vi "Sensirion SHT25 - VISA test.vi"() -> ()   [LabVIEW 2012]
uses:
  Sensirion SHT25 - measurement resolution.ctl
panel:
  in  "Reset":bool
  in  "resolution":T1 items=["RH 12, T 14"=0, "RH 8, T 12"=1, "RH 10, T 13"=128, "RH 11, T 11"=129]
  out "user register":u8 format="%08b"
  out "IO pins (initially)":string
  out "Data Chart":cluster{"temperature":dbl, "humidity":dbl}(graph)
  out "temperature":dbl format="%.2f"
  out "humidity":dbl format="%.2f"
  in  "Stop":bool
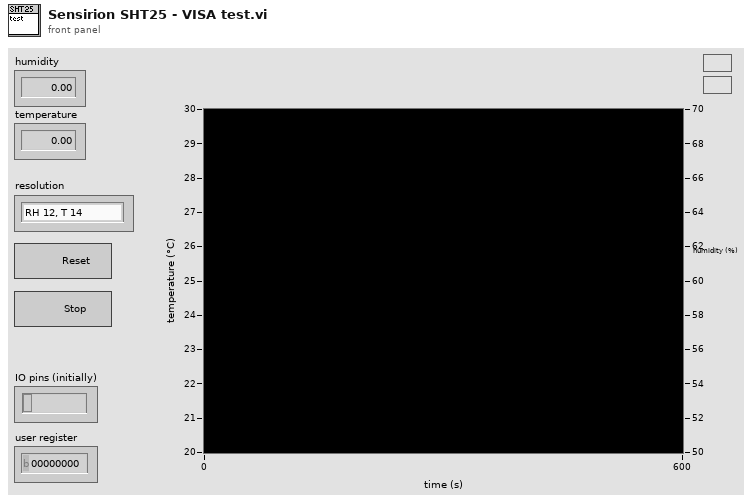
[diagram p1: front panel]
types:
  T1 = typedef "Sensirion SHT25 - measurement resolution.ctl" = u8
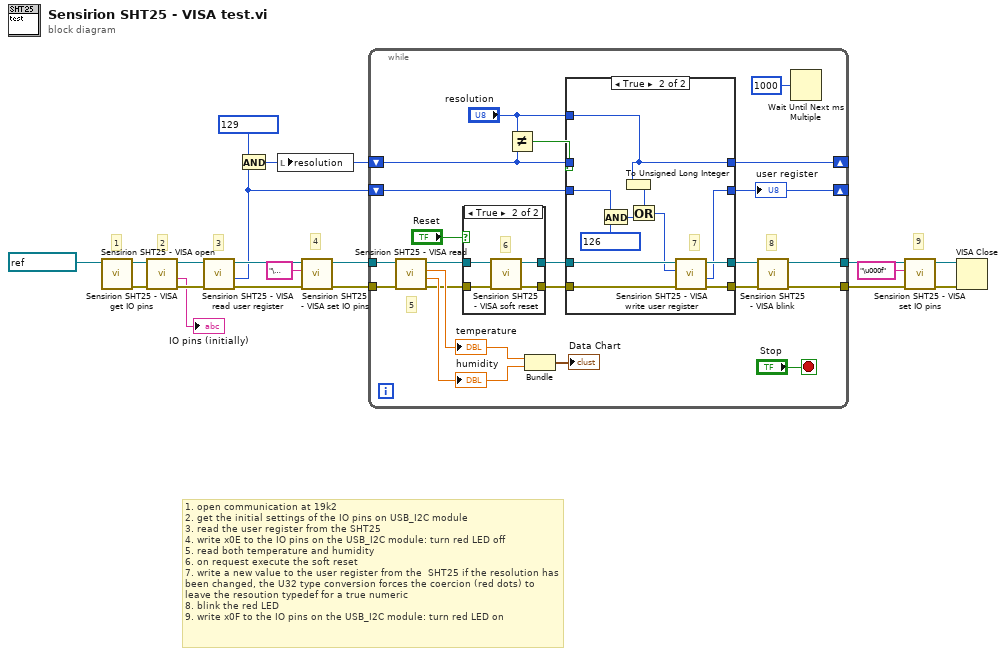
[diagram p0: block diagram]
diagram:
  # "1. open communication at 19k2\n2. get the initial settings of the IO pins on USB_I2C module\n3. read the user register from the SHT25\n4. write x0E to the IO pins on the USB_I2C module: turn red LED off\n5. read both temperature and humidity\n6. on request execute the soft reset\n7. write a new value to the user register from the  SHT25 if the resolution has been changed, the U32 type conversion forces the coercion (red dots) to leave the resoution typedef for a true numeric\n8. blink the red LED\n9. write x0F to the IO pins on the USB_I2C module: turn red LED on"
  # "9"
  # "4"
  # "3"
  # "2"
  # "1"
  n1 = call "Sensirion SHT25 - VISA open.vi"("VISA in"=refnum<visa-resource-name> "COM12") -> ("Error Out"=w15:errorcluster, "VISA out"=w16:refnum<visa-resource-name>)  [unwired: 9 in]
  n2 = call "Sensirion SHT25 - VISA get IO pins.vi"("Error In"=w15, "VISA in"=w16) -> ("Error Out"=w6:errorcluster, "read buffer"=→"IO pins (initially)":string, "VISA out"=w8:refnum<visa-resource-name>)  [unwired: 7 in]
  n3 = call "Sensirion SHT25 - VISA read user register.vi"("Error In"=w6, "VISA in"=w8) -> ("Error Out"=w5:errorcluster, "user register"=w1:u8, "VISA out"=w7:refnum<visa-resource-name>)  [unwired: 7 in]
  n4 = And(x=u8 129 ("y"), y=w1) -> (x .and. y?=w2:u8)
  n5 = local write "resolution"(w2) -> ()
  n6 = call "Sensirion SHT25 - VISA set IO pins.vi"("Error In"=w5, "I/O pins"="\u000e", "VISA in"=w7) -> ("Error Out"=w17:errorcluster, "VISA out"=w18:refnum<visa-resource-name>)  [unwired: 6 in, 1 out]
  n7 = while {
    tunnel: w18 -> [w40]
    tunnel: [w21] -> w12
    tunnel: w17 -> [w39]
    tunnel: [w20] -> w11
    shift-right: [w29] -> _
    shift-left: w2 -> [w30]
    shift-right: [w26] -> _
    shift-left: w1 -> [w27]
    stop <- "Stop" stop-if-true
    # "8"
    # "5"
    n8 = call "Sensirion SHT25 - VISA read.vi"("Error In"=w39, "VISA in"=w40) -> ("Error Out"=w24:errorcluster, "humidity"=w35:dbl, "temperature"=w36:dbl, "VISA out"=w25:refnum<visa-resource-name>)  [unwired: 6 in]
    "humidity" <- w35
    "temperature" <- w36
    n9 = case shown="True" "Reset" {
      tunnel: w25 -> [w58 w61]
      tunnel: [w58 w60] -> w33
      tunnel: w24 -> [w57 w62]
      tunnel: [w57 w59] -> w32
      frame False {
      }
      frame True {
        # "6"
        n10 = call "Sensirion SHT25 - VISA soft reset.vi"("Error In"=w62, "VISA in"=w61) -> ("Error Out"=w59:errorcluster, "VISA out"=w60:refnum<visa-resource-name>)  [unwired: 7 in, 1 out]
      }
    }
    n11 = Not Equal?(x="resolution", y=w30) -> (x != y?=w31:bool)
    n12 = Bundle("temperature"=w36, "humidity"=w35) -> (→"Data Chart":cluster{"temperature":dbl, "humidity":dbl})  [unwired: 1 in]
    n13 = case shown="True" w31 {
      tunnel: w33 -> [w45 w55]
      tunnel: [w45 w53] -> w23
      tunnel: w32 -> [w44 w56]
      tunnel: [w44 w54] -> w22
      tunnel: w30 -> [w43 _]
      tunnel: [w43 w51] -> w29
      tunnel: "resolution" -> [_ w51]
      tunnel: w27 -> [w42 w49]
      tunnel: [w42 w48] -> w26
      frame False {
      }
      frame True {
        # "7"
        n14 = And(x=w49, y=u8 126) -> (x .and. y?=w46:u8)
        n15 = To Unsigned Long Integer(number=w51) -> (unsigned 32bit integer=w47:u32)
        n16 = Or(x=w47, y=w46) -> (x .or. y?=w50:u32)
        n17 = call "Sensirion SHT25 - VISA write user register.vi"("Error In"=w56, "user register (in)"=w50, "VISA in"=w55) -> ("Error Out"=w54:errorcluster, "user register (out)"=w48:u8, "VISA out"=w53:refnum<visa-resource-name>)  [unwired: 6 in]
      }
    }
    "user register" <- w26
    n18 = call "Sensirion SHT25 - VISA blink.vi"("Error In"=w22, "VISA in"=w23) -> ("Error Out"=w20:errorcluster, "VISA out"=w21:refnum<visa-resource-name>)  [unwired: 8 in]
    n19 = Wait Until Next ms Multiple(millisecond multiple=u32 1000) -> ()  [unwired: 1 out]
  }
  n20 = call "Sensirion SHT25 - VISA set IO pins.vi"("Error In"=w11, "I/O pins"="\u000f", "VISA in"=w12) -> ("Error Out"=w9:errorcluster, "VISA out"=w10:refnum<visa-resource-name>)  [unwired: 6 in, 1 out]
  n21 = VISA Close(VISA resource name=w10, error in (no error)=w9) -> ()  [unwired: 1 out]
